vi "ConsumeNumber.vi"(8 "error in (no error)":errorcluster, 11 "TransformTokenizer in":refnum<class "TransformTokenizer.lvclass">) -> (0 "error out":errorcluster, 3 "TransformTokenizer out":refnum<class "TransformTokenizer.lvclass">)   [LabVIEW 2019, in "TransformTokenizer.lvclass"]
uses:
  TransformTokenizer.lvclass
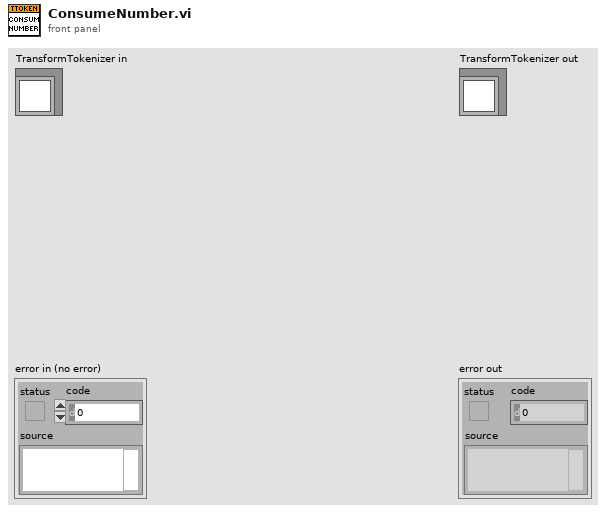
[diagram p1: front panel]
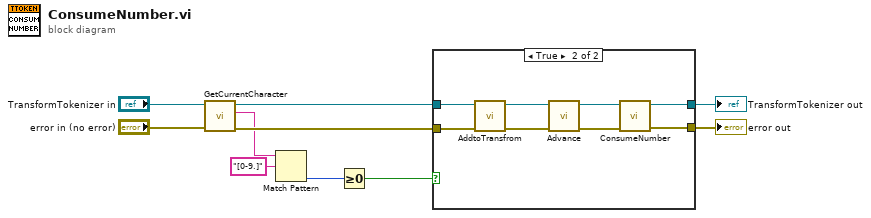
[diagram p0: block diagram]
diagram:
  n1 = call "GetCurrentCharacter.vi"("error in (no error)"="error in (no error)", "TransformTokenizer in"="TransformTokenizer in") -> ("error out"=w8:errorcluster, "Character"=w4:string, "TransformTokenizer out"=w9:refnum<class "TransformTokenizer.lvclass">)  [unwired: 7 in]
  n2 = Match Pattern(string=w4, regular expression="[0-9.]") -> (offset past match=w2:i32)  [unwired: 1 in, 3 out]
  n3 = Greater Or Equal To 0?(x=w2) -> (x >= 0?=w1:bool)
  n4 = case shown="True" w1 {
    tunnel: w9 -> [w12 w20]
    tunnel: w8 -> [w11 w19]
    tunnel: [w12 w14] -> w7
    tunnel: [w11 w13] -> w5
    frame False {
    }
    frame True {
      n5 = call "AddtoTransfrom.vi"("error in (no error)"=w19, "TransformTokenizer in"=w20) -> ("error out"=w17:errorcluster, "TransformTokenizer out"=w18:refnum<class "TransformTokenizer.lvclass">)  [unwired: 8 in]
      n6 = call "Advance.vi"("error in (no error)"=w17, "TransformTokenizer in"=w18) -> ("error out"=w15:errorcluster, "TransformTokenizer out"=w16:refnum<class "TransformTokenizer.lvclass">)  [unwired: 8 in]
      n7 = call "ConsumeNumber.vi"("error in (no error)"=w15, "TransformTokenizer in"=w16) -> ("error out"=w13:errorcluster, "TransformTokenizer out"=w14:refnum<class "TransformTokenizer.lvclass">)  [unwired: 8 in]
    }
  }
  "error out" <- w5
  "TransformTokenizer out" <- w7
